vi "Autonomous Independent.vi"   [LabVIEW 2017]
doc: "This VI is called when autonomous begins, and will automatically be terminated when autonomous ends. You can carry out timed or sensor driven robot movement independently without needing to return to the caller."
uses:
  <vilib>/Rock Robotics/WPI/Utilities/WPI_GetSetVariantRefNum.vi
  <vilib>/Rock Robotics/Network Tables/NT Read String.vi
  <vilib>/Rock Robotics/Network Tables/NT Write Numeric Array.vi
  <vilib>/Rock Robotics/WPI/RobotDrive/WPI_RobotDriveArcadeDrive_Standard(NoSaturation).vi
panel:
  # "Be sure to right-click and choose Data Operations>>Make Current Value default if you want to save the array values with the VI"
types:
  T1 = typedef "WPI_JoystickDevRef.ctl" = cluster{"Device":T2}
  T2 = typedef "WPI_JoystickDeviceEnum.ctl" = enum16{"USB 0", "USB 1", "USB 2", "USB 3", "USB 4", "USB 5"}
  T3 = typedef "WPI_MotorControlDeviceRef.ctl" = cluster{"DeviceStatus":errorcluster, "Type":T4, "PWM":cluster{"PWM Channel":T5, "DeadBand":T6}, "CAN":cluster{"Device Number":u8, "SetOutput VI Ref":variant, "GetOutput VI Ref":variant, "Enable VI Ref":variant, "Disable VI Ref":variant, "Data":variant}, "Invert":bool, "DIO PWM":cluster{"PWM \"Enable\" Channel":T5, "DIOChannel":T7, "PWM Rate":dbl}}
  T4 = typedef "WPI_MotorControlType.ctl" = enum16{"PWM", "CAN", "DIO PWM"}
  T5 = typedef "FPGA_DIOPWMChannel.ctl" = enum8{"PWM 0", "PWM 1", "PWM 2", "PWM 3", "PWM 4", "PWM 5", "PWM 6", "PWM 7", "PWM 8", "PWM 9", "PWM MXP 0", "PWM MXP 1", "PWM MXP 2", "PWM MXP 3", "PWM MXP 4", "PWM MXP 5", "PWM MXP 6", "PWM MXP 7", "PWM MXP 8", "PWM MXP 9", "Invalid"}
  T6 = typedef "WPI_PWMDeadband.ctl" = cluster{"Name":string, "maxPositivePwm":i32, "minPositivePwm":i32, "centerPwm":i32, "maxNegativePwm":i32, "minNegativePwm":i32, "angularRange":u16}
  T7 = typedef "FPGA_DIOChannel.ctl" = enum8{"DIO 0", "DIO 1", "DIO 2", "DIO 3", "DIO 4", "DIO 5", "DIO 6", "DIO 7", "DIO 8", "DIO 9", "DIO MXP 0", "DIO MXP 1", "DIO MXP 2", "DIO MXP 3", "DIO MXP 4", "DIO MXP 5", "DIO MXP 6", "DIO MXP 7", "DIO MXP 8", "DIO MXP 9", "DIO MXP 10", "DIO MXP 11", "DIO MXP 12", "DIO MXP 13", "DIO MXP 14", "DIO MXP 15", "SPI Port CS1", "SPI Port CS2", "SPI Port CS3", "SPI Port MISO", "SPI Port MOSI", "Invalid"}
  T8 = typedef "WPI_RobotDriveDevRef.ctl" = cluster{"DevStatus":errorcluster, "Motors[]":T3[], "Square Inputs":bool, "Max Output":dbl}
  T9 = typedef "WPI_SwitchDevRef.ctl" = cluster{"DevStatus":errorcluster, "DIO Channel":T7, "CntIndex":T10, "Normally Closed":bool}
  T10 = typedef "FPGA_CounterCtrSystemIndex.ctl" = enum8{"Ctr 0", "Ctr 1", "Ctr 2", "Ctr 3", "Ctr 4", "Ctr 5", "Ctr 6", "Ctr 7", "Invalid"}
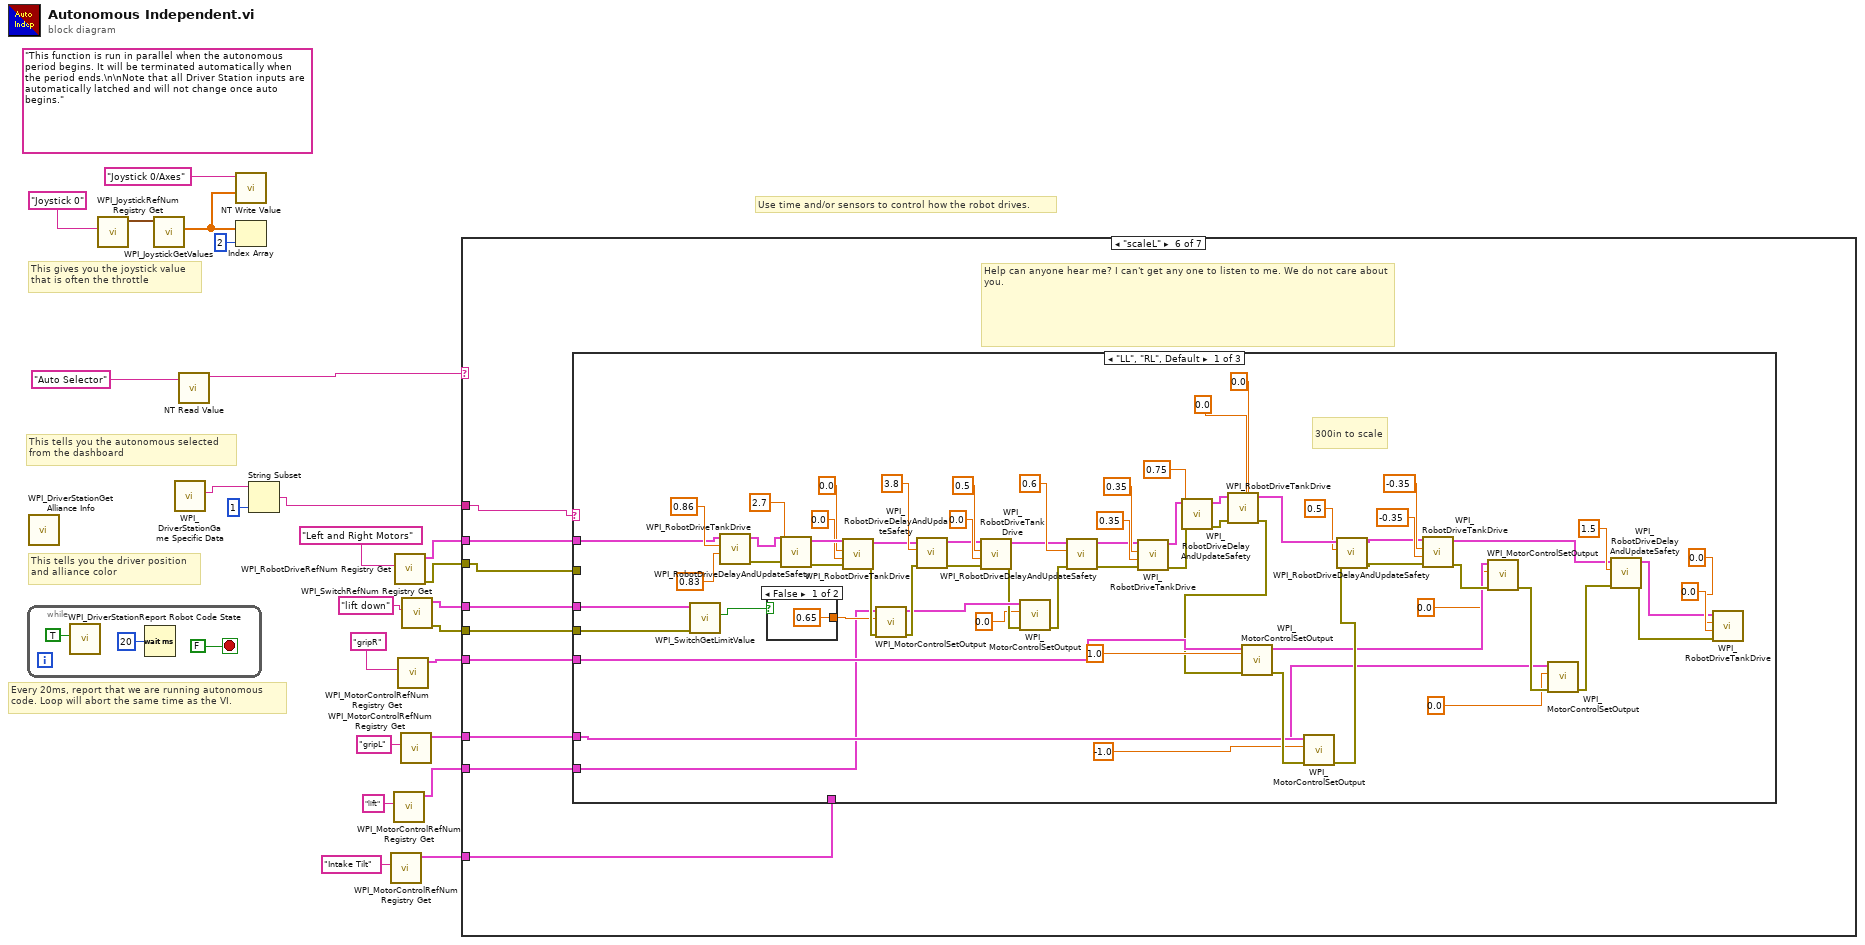
[diagram p0: block diagram]
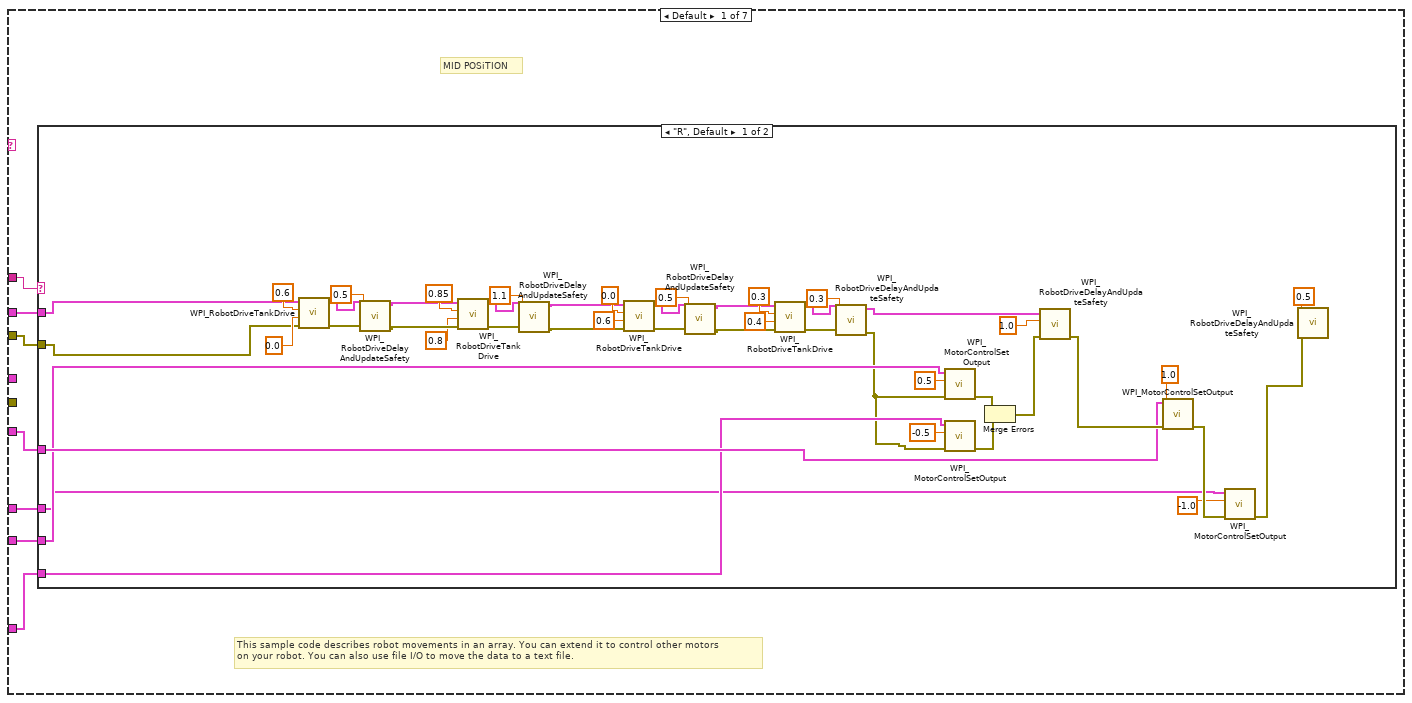
[diagram p2: hidden frame]
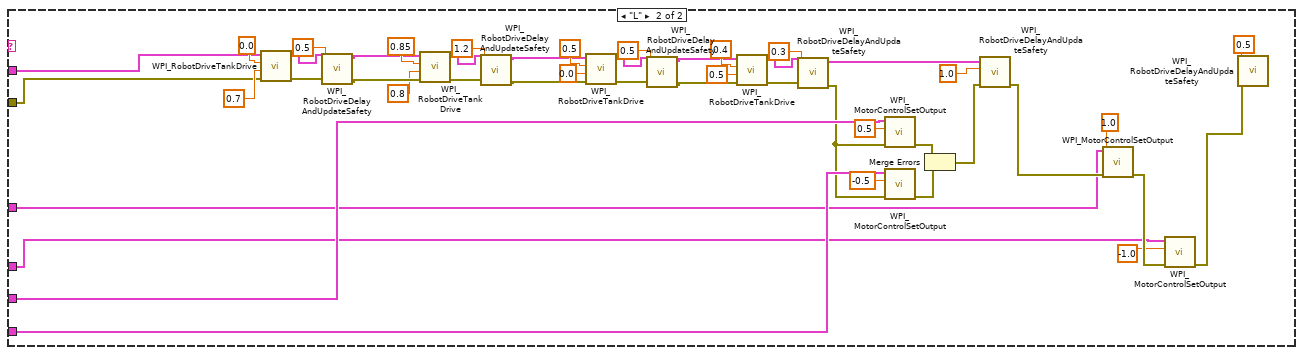
[diagram p3: hidden frame]
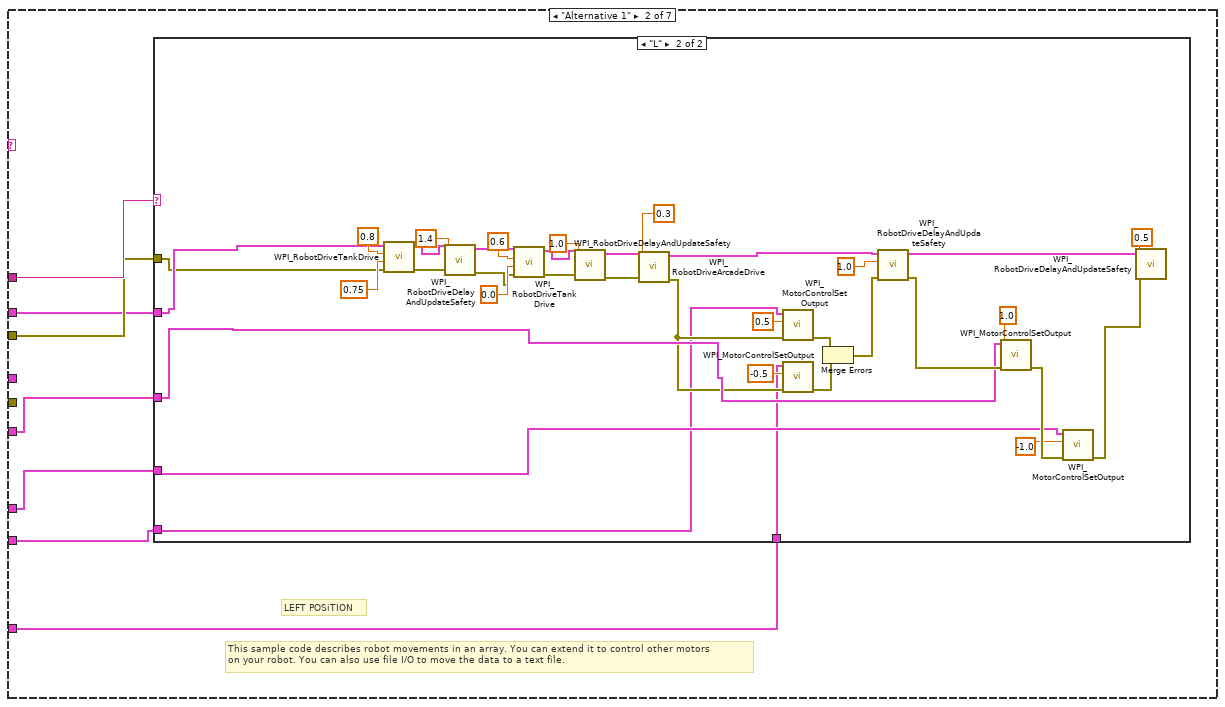
[diagram p4: hidden frame]
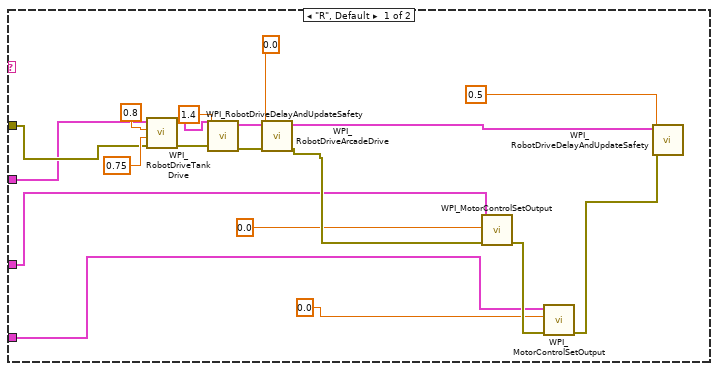
[diagram p5: hidden frame]
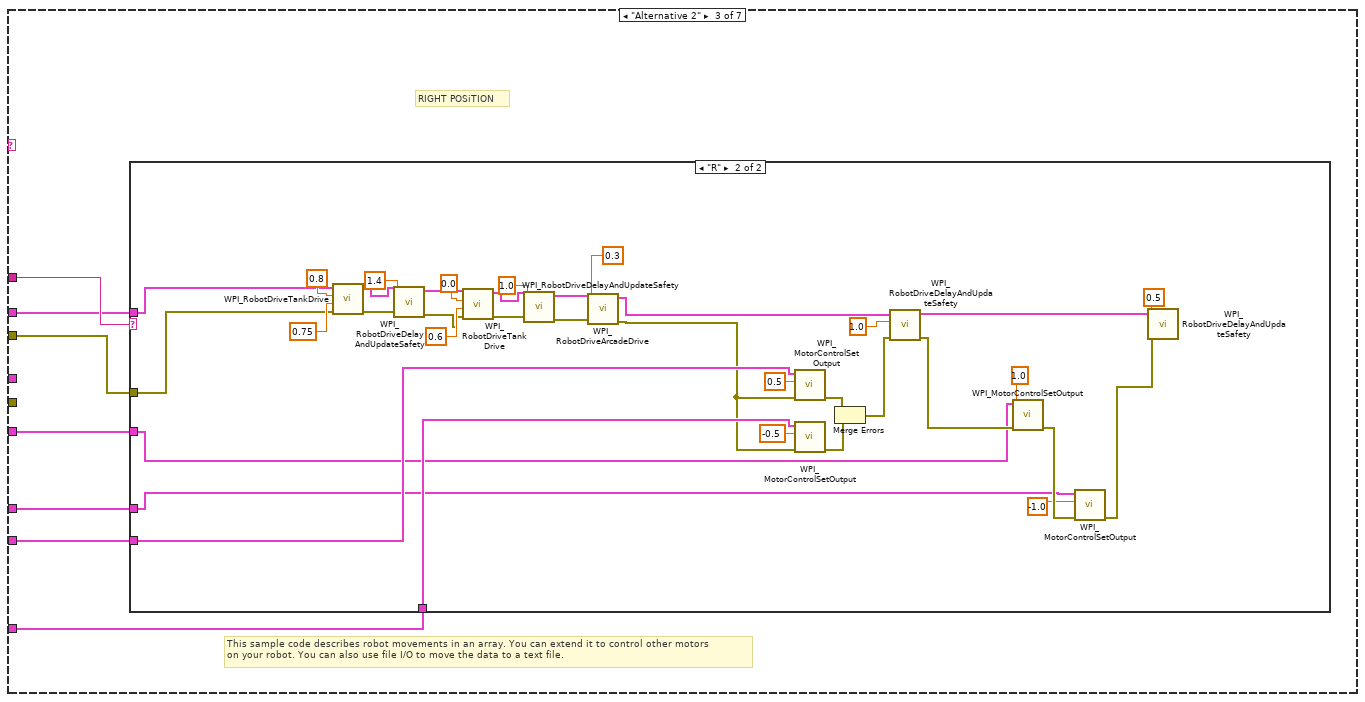
[diagram p6: hidden frame]
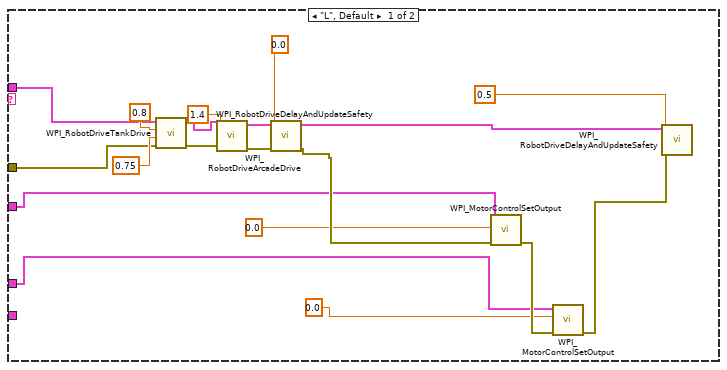
[diagram p7: hidden frame]
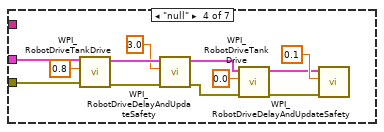
[diagram p8: hidden frame]
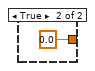
[diagram p10: hidden frame]
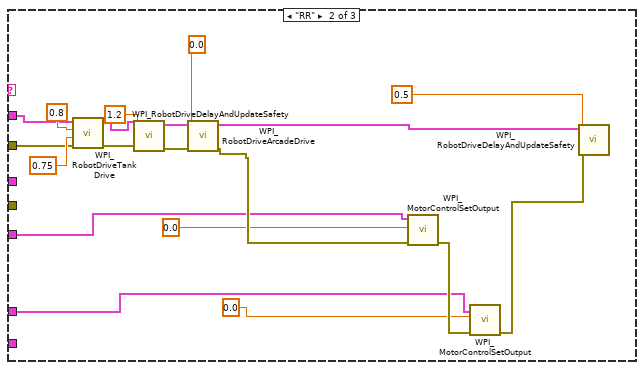
[diagram p11: hidden frame]
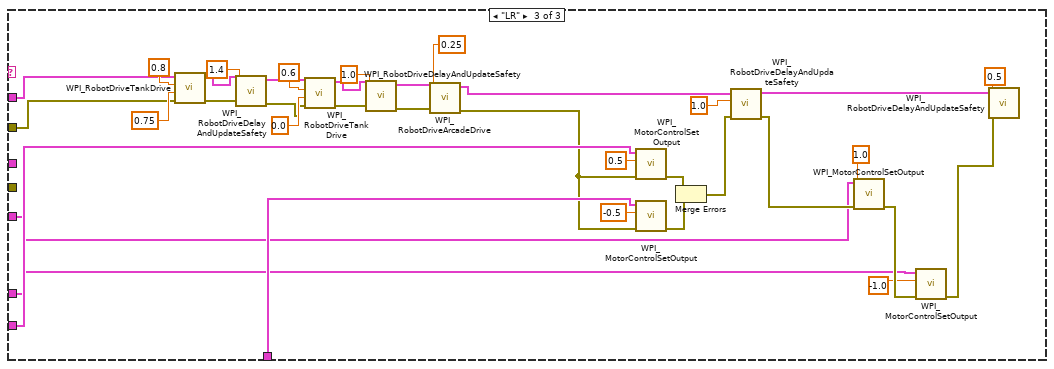
[diagram p12: hidden frame]
diagram:
  (unwired) "This function is run in parallel when the autonomous period begins. It will be terminated automatically when the period ends.\n\nNote that all Driver Station inputs are automatically latched and will not change once auto begins."
  # "This tells you the autonomous selected\nfrom the dashboard"
  # "Every 20ms, report that we are running autonomous\ncode. Loop will abort the same time as the VI."
  # "This gives you the joystick value\nthat is often the throttle"
  # "Use time and/or sensors to control how the robot drives."
  # "This tells you the driver position\nand alliance color"
  n1 = while {
    stop <- FALSE stop-if-true
    n2 = call <vilib>:"WPI_DriverStationReport Robot Code State.vi"("Autonomous"=TRUE) -> ()  [unwired: 10 in, 1 out]
    n3 = Wait (ms)(milliseconds to wait=u32 20) -> ()  [unwired: 1 out]
  }
  n4 = call <vilib>:"WPI_DriverStationGet Alliance Info.vi"() -> ()  [unwired: 12 out]
  n5 = call <vilib>:"WPI_JoystickRefNum Registry Get.vi"("refnum name"="Joystick 0") -> ("JoystickDevRef"=w23:T1)  [unwired: 1 in, 9 out]
  n6 = call <vilib>:"WPI_JoystickGetValues.vi"("JoystickDevRef"=w23) -> ("Axes"=w19:dbl[])  [unwired: 6 in, 4 out]
  n7 = call <vilib>:"WPI_DriverStationGame Specific Data.vi"() -> ("Game Specific Data"=w17:string)  [unwired: 11 in]
  n8 = call-poly <vilib>:"NT Read Value.vi"("Name"="Auto Selector") -> ("String"=w20:string)  [unwired: 9 in, 1 out]
  n9 = call-poly <vilib>:"NT Write Value.vi"("Numeric Array"=w19, "Name"="Joystick 0/Axes") -> ()  [unwired: 9 in, 1 out]
  n10 = Index Array(array=w19, index=2) -> ()  [unwired: 1 out]
  n11 = String Subset(string=w17, length (rest)=1 ("length (rest)")) -> (substring=w15:string)  [unwired: 1 in]
  n12 = call <vilib>:"WPI_MotorControlRefNum Registry Get.vi"("refnum name"="Intake Tilt") -> ("MotorControlDevRef"=w1:T3)  [unwired: 9 in, 1 out]
  n13 = call <vilib>:"WPI_MotorControlRefNum Registry Get.vi"("refnum name"="lift") -> ("MotorControlDevRef"=w3:T3)  [unwired: 9 in, 1 out]
  n14 = call <vilib>:"WPI_RobotDriveRefNum Registry Get.vi"("refnum name"="Left and Right Motors") -> ("error out"=w13:errorcluster, "RobotDriveDevRef"=w8:T8)  [unwired: 1 in, 8 out]
  n15 = call <vilib>:"WPI_MotorControlRefNum Registry Get.vi"("refnum name"="gripR") -> ("MotorControlDevRef"=w11:T3)  [unwired: 9 in, 1 out]
  n16 = call <vilib>:"WPI_MotorControlRefNum Registry Get.vi"("refnum name"="gripL") -> ("MotorControlDevRef"=w9:T3)  [unwired: 9 in, 1 out]
  n17 = call <vilib>:"WPI_SwitchRefNum Registry Get.vi"("refnum name"="lift down") -> ("error out"=w5:errorcluster, "SwitchDevRef"=w4:T9)  [unwired: 9 in]
  n18 = case shown="\"scaleL\"" w20 {
    tunnel: w15 -> [w34 w133 w195 _ _ w271 _]
    tunnel: w13 -> [w33 w132 w194 w261 _ w264 _]
    tunnel: w11 -> [w32 w131 w193 _ _ w268 _]
    tunnel: w9 -> [w31 w130 w192 _ _ w269 _]
    tunnel: w8 -> [w30 w129 w191 w262 _ w270 _]
    tunnel: w5 -> [_ _ _ _ _ w267 _]
    tunnel: w4 -> [_ _ _ _ _ w266 _]
    tunnel: w3 -> [w28 w127 w190 _ _ w265 _]
    tunnel: w1 -> [w29 w128 w189 _ _ w263 _]
    frame Default {
      # "MID POSiTION"
      # "This sample code describes robot movements in an array. You can extend it to control other motors\non your robot. You can also use file I/O to move the data to a text file."
      n19 = case shown="\"R\", Default" w34 {
        tunnel: w33 -> [w75 w95]
        tunnel: w32 -> [w39 w82]
        tunnel: w31 -> [w36 w81]
        tunnel: w30 -> [w53 w94]
        tunnel: w29 -> [w37 w89]
        tunnel: w28 -> [w38 w93]
        frame "R", Default {
          n20 = call <vilib>:"WPI_RobotDriveTankDrive.vi"("error in (no error)"=w75, "Right axis value"=0.0 ("Y axis value"), "Left axis value"=0.6 ("X axis value"), "RobotDriveDevRef"=w53) -> ("error out"=w79:errorcluster, "RobotDriveDevRef"=w78:T8)  [unwired: 5 in, 1 out]
          n21 = call <vilib>:"WPI_RobotDriveDelayAndUpdateSafety.vi"("error in (no error)"=w79, "Delay (s)"=0.5, "RobotDriveDevRef"=w78) -> ("error out"=w69:errorcluster, "RobotDriveDevRef 2"=w70:T8)  [unwired: 7 in]
          n22 = call <vilib>:"WPI_RobotDriveTankDrive.vi"("error in (no error)"=w69, "Right axis value"=0.8, "Left axis value"=0.85 ("X axis value"), "RobotDriveDevRef"=w70) -> ("error out"=w73:errorcluster, "RobotDriveDevRef"=w72:T8)  [unwired: 5 in, 1 out]
          n23 = call <vilib>:"WPI_RobotDriveDelayAndUpdateSafety.vi"("error in (no error)"=w73, "Delay (s)"=1.1, "RobotDriveDevRef"=w72) -> ("error out"=w62:errorcluster, "RobotDriveDevRef 2"=w63:T8)  [unwired: 7 in]
          n24 = call <vilib>:"WPI_RobotDriveTankDrive.vi"("error in (no error)"=w62, "Right axis value"=0.6, "Left axis value"=0.0 ("X axis value"), "RobotDriveDevRef"=w63) -> ("error out"=w66:errorcluster, "RobotDriveDevRef"=w65:T8)  [unwired: 5 in, 1 out]
          n25 = call <vilib>:"WPI_RobotDriveDelayAndUpdateSafety.vi"("error in (no error)"=w66, "Delay (s)"=0.5, "RobotDriveDevRef"=w65) -> ("error out"=w55:errorcluster, "RobotDriveDevRef 2"=w56:T8)  [unwired: 7 in]
          n26 = call <vilib>:"WPI_RobotDriveTankDrive.vi"("error in (no error)"=w55, "Right axis value"=0.4, "Left axis value"=0.3 ("X axis value"), "RobotDriveDevRef"=w56) -> ("error out"=w59:errorcluster, "RobotDriveDevRef"=w58:T8)  [unwired: 5 in, 1 out]
          n27 = call <vilib>:"WPI_RobotDriveDelayAndUpdateSafety.vi"("error in (no error)"=w59, "Delay (s)"=0.3, "RobotDriveDevRef"=w58) -> ("error out"=w35:errorcluster, "RobotDriveDevRef 2"=w40:T8)  [unwired: 7 in]
          n28 = call <vilib>:"WPI_MotorControlSetOutput.vi"("error in (no error)"=w35, "Output"=0.5, "MotorControlDevRef"=w38) -> ("error out"=w43:errorcluster)  [unwired: 6 in, 2 out]
          n29 = call <vilib>:"WPI_MotorControlSetOutput.vi"("error in (no error)"=w35, "Output"=-0.5, "MotorControlDevRef"=w37) -> ("error out"=w44:errorcluster)  [unwired: 6 in, 2 out]
          n30 = Merge Errors(w43, w44) -> (w42:errorcluster)
          n31 = call <vilib>:"WPI_RobotDriveDelayAndUpdateSafety.vi"("error in (no error)"=w42, "Delay (s)"=1.0, "RobotDriveDevRef"=w40) -> ("error out"=w41:errorcluster)  [unwired: 7 in, 1 out]
          n32 = call <vilib>:"WPI_MotorControlSetOutput.vi"("error in (no error)"=w41, "Output"=1.0, "MotorControlDevRef"=w39) -> ("error out"=w51:errorcluster)  [unwired: 6 in, 2 out]
          n33 = call <vilib>:"WPI_MotorControlSetOutput.vi"("error in (no error)"=w51, "Output"=-1.0, "MotorControlDevRef"=w36) -> ("error out"=w50:errorcluster)  [unwired: 6 in, 2 out]
          n34 = call <vilib>:"WPI_RobotDriveDelayAndUpdateSafety.vi"("error in (no error)"=w50, "Delay (s)"=0.5) -> ()  [unwired: 8 in, 2 out]
        }
        frame "L" {
          n35 = call <vilib>:"WPI_RobotDriveTankDrive.vi"("error in (no error)"=w95, "Right axis value"=0.7 ("Y axis value"), "Left axis value"=0.0 ("X axis value"), "RobotDriveDevRef"=w94) -> ("error out"=w122:errorcluster, "RobotDriveDevRef"=w121:T8)  [unwired: 5 in, 1 out]
          n36 = call <vilib>:"WPI_RobotDriveDelayAndUpdateSafety.vi"("error in (no error)"=w122, "Delay (s)"=0.5, "RobotDriveDevRef"=w121) -> ("error out"=w111:errorcluster, "RobotDriveDevRef 2"=w112:T8)  [unwired: 7 in]
          n37 = call <vilib>:"WPI_RobotDriveTankDrive.vi"("error in (no error)"=w111, "Right axis value"=0.8, "Left axis value"=0.85 ("X axis value"), "RobotDriveDevRef"=w112) -> ("error out"=w115:errorcluster, "RobotDriveDevRef"=w114:T8)  [unwired: 5 in, 1 out]
          n38 = call <vilib>:"WPI_RobotDriveDelayAndUpdateSafety.vi"("error in (no error)"=w115, "Delay (s)"=1.2, "RobotDriveDevRef"=w114) -> ("error out"=w104:errorcluster, "RobotDriveDevRef 2"=w105:T8)  [unwired: 7 in]
          n39 = call <vilib>:"WPI_RobotDriveTankDrive.vi"("error in (no error)"=w104, "Right axis value"=0.0, "Left axis value"=0.5 ("X axis value"), "RobotDriveDevRef"=w105) -> ("error out"=w108:errorcluster, "RobotDriveDevRef"=w107:T8)  [unwired: 5 in, 1 out]
          n40 = call <vilib>:"WPI_RobotDriveDelayAndUpdateSafety.vi"("error in (no error)"=w108, "Delay (s)"=0.5, "RobotDriveDevRef"=w107) -> ("error out"=w97:errorcluster, "RobotDriveDevRef 2"=w98:T8)  [unwired: 7 in]
          n41 = call <vilib>:"WPI_RobotDriveTankDrive.vi"("error in (no error)"=w97, "Right axis value"=0.5, "Left axis value"=0.4 ("X axis value"), "RobotDriveDevRef"=w98) -> ("error out"=w101:errorcluster, "RobotDriveDevRef"=w100:T8)  [unwired: 5 in, 1 out]
          n42 = call <vilib>:"WPI_RobotDriveDelayAndUpdateSafety.vi"("error in (no error)"=w101, "Delay (s)"=0.3, "RobotDriveDevRef"=w100) -> ("error out"=w87:errorcluster, "RobotDriveDevRef 2"=w91:T8)  [unwired: 7 in]
          n43 = call <vilib>:"WPI_MotorControlSetOutput.vi"("error in (no error)"=w87, "Output"=0.5, "MotorControlDevRef"=w93) -> ("error out"=w85:errorcluster)  [unwired: 6 in, 2 out]
          n44 = call <vilib>:"WPI_MotorControlSetOutput.vi"("error in (no error)"=w87, "Output"=-0.5, "MotorControlDevRef"=w89) -> ("error out"=w86:errorcluster)  [unwired: 6 in, 2 out]
          n45 = Merge Errors(w85, w86) -> (w84:errorcluster)
          n46 = call <vilib>:"WPI_RobotDriveDelayAndUpdateSafety.vi"("error in (no error)"=w84, "Delay (s)"=1.0, "RobotDriveDevRef"=w91) -> ("error out"=w83:errorcluster)  [unwired: 7 in, 1 out]
          n47 = call <vilib>:"WPI_MotorControlSetOutput.vi"("error in (no error)"=w83, "Output"=1.0, "MotorControlDevRef"=w82) -> ("error out"=w124:errorcluster)  [unwired: 6 in, 2 out]
          n48 = call <vilib>:"WPI_MotorControlSetOutput.vi"("error in (no error)"=w124, "Output"=-1.0, "MotorControlDevRef"=w81) -> ("error out"=w123:errorcluster)  [unwired: 6 in, 2 out]
          n49 = call <vilib>:"WPI_RobotDriveDelayAndUpdateSafety.vi"("error in (no error)"=w123, "Delay (s)"=0.5) -> ()  [unwired: 8 in, 2 out]
        }
      }
    }
    frame "Alternative 1" {
      # "LEFT POSiTION"
      # "This sample code describes robot movements in an array. You can extend it to control other motors\non your robot. You can also use file I/O to move the data to a text file."
      n50 = case shown="\"L\"" w133 {
        tunnel: w132 -> [w137 w172]
        tunnel: w131 -> [w136 w158]
        tunnel: w130 -> [w135 w156]
        tunnel: w129 -> [w134 w173]
        tunnel: w128 -> [_ w155]
        tunnel: w127 -> [_ w154]
        frame "R", Default {
          n51 = call <vilib>:"WPI_RobotDriveTankDrive.vi"("error in (no error)"=w137, "Right axis value"=0.75 ("Y axis value"), "Left axis value"=0.8 ("X axis value"), "RobotDriveDevRef"=w134) -> ("error out"=w143:errorcluster, "RobotDriveDevRef"=w142:T8)  [unwired: 5 in, 1 out]
          n52 = call <vilib>:"WPI_RobotDriveDelayAndUpdateSafety.vi"("error in (no error)"=w143, "Delay (s)"=1.4, "RobotDriveDevRef"=w142) -> ("error out"=w151:errorcluster, "RobotDriveDevRef 2"=w150:T8)  [unwired: 7 in]
          n53 = call-poly <vilib>:"WPI_RobotDriveArcadeDrive.vi"("error in (no error)"=w151, "Y axis value"=0.0, "RobotDriveDevRef"=w150) -> ("error out"=w145:errorcluster, "RobotDriveDevRef"=w148:T8)  [unwired: 6 in, 1 out]
          n54 = call <vilib>:"WPI_MotorControlSetOutput.vi"("error in (no error)"=w145, "Output"=0.0, "MotorControlDevRef"=w136) -> ("error out"=w146:errorcluster)  [unwired: 6 in, 2 out]
          n55 = call <vilib>:"WPI_MotorControlSetOutput.vi"("error in (no error)"=w146, "Output"=0.0, "MotorControlDevRef"=w135) -> ("error out"=w144:errorcluster)  [unwired: 6 in, 2 out]
          n56 = call <vilib>:"WPI_RobotDriveDelayAndUpdateSafety.vi"("error in (no error)"=w144, "Delay (s)"=0.5, "RobotDriveDevRef"=w148) -> ()  [unwired: 7 in, 2 out]
        }
        frame "L" {
          n57 = call <vilib>:"WPI_RobotDriveTankDrive.vi"("error in (no error)"=w172, "Right axis value"=0.75 ("Y axis value"), "Left axis value"=0.8 ("X axis value"), "RobotDriveDevRef"=w173) -> ("error out"=w186:errorcluster, "RobotDriveDevRef"=w185:T8)  [unwired: 5 in, 1 out]
          n58 = call <vilib>:"WPI_RobotDriveDelayAndUpdateSafety.vi"("error in (no error)"=w186, "Delay (s)"=1.4, "RobotDriveDevRef"=w185) -> ("error out"=w176:errorcluster, "RobotDriveDevRef 2"=w177:T8)  [unwired: 7 in]
          n59 = call <vilib>:"WPI_RobotDriveTankDrive.vi"("error in (no error)"=w176, "Right axis value"=0.0 ("Y axis value"), "Left axis value"=0.6 ("X axis value"), "RobotDriveDevRef"=w177) -> ("error out"=w181:errorcluster, "RobotDriveDevRef"=w180:T8)  [unwired: 5 in, 1 out]
          n60 = call <vilib>:"WPI_RobotDriveDelayAndUpdateSafety.vi"("error in (no error)"=w181, "Delay (s)"=1.0, "RobotDriveDevRef"=w180) -> ("error out"=w174:errorcluster, "RobotDriveDevRef 2"=w175:T8)  [unwired: 7 in]
          n61 = call-poly <vilib>:"WPI_RobotDriveArcadeDrive.vi"("error in (no error)"=w174, "Y axis value"=0.3, "RobotDriveDevRef"=w175) -> ("error out"=w157:errorcluster, "RobotDriveDevRef"=w159:T8)  [unwired: 6 in, 1 out]
          n62 = call <vilib>:"WPI_MotorControlSetOutput.vi"("error in (no error)"=w157, "Output"=0.5, "MotorControlDevRef"=w154) -> ("error out"=w162:errorcluster)  [unwired: 6 in, 2 out]
          n63 = call <vilib>:"WPI_MotorControlSetOutput.vi"("error in (no error)"=w157, "Output"=-0.5, "MotorControlDevRef"=w155) -> ("error out"=w163:errorcluster)  [unwired: 6 in, 2 out]
          n64 = Merge Errors(w162, w163) -> (w161:errorcluster)
          n65 = call <vilib>:"WPI_RobotDriveDelayAndUpdateSafety.vi"("error in (no error)"=w161, "Delay (s)"=1.0, "RobotDriveDevRef"=w159) -> ("error out"=w160:errorcluster, "RobotDriveDevRef 2"=w153:T8)  [unwired: 7 in]
          n66 = call <vilib>:"WPI_MotorControlSetOutput.vi"("error in (no error)"=w160, "Output"=1.0, "MotorControlDevRef"=w158) -> ("error out"=w170:errorcluster)  [unwired: 6 in, 2 out]
          n67 = call <vilib>:"WPI_MotorControlSetOutput.vi"("error in (no error)"=w170, "Output"=-1.0, "MotorControlDevRef"=w156) -> ("error out"=w169:errorcluster)  [unwired: 6 in, 2 out]
          n68 = call <vilib>:"WPI_RobotDriveDelayAndUpdateSafety.vi"("error in (no error)"=w169, "Delay (s)"=0.5, "RobotDriveDevRef"=w153) -> ()  [unwired: 7 in, 2 out]
        }
      }
    }
    frame "Alternative 2" {
      # "RIGHT POSiTION"
      # "This sample code describes robot movements in an array. You can extend it to control other motors\non your robot. You can also use file I/O to move the data to a text file."
      n69 = case shown="\"R\"" w195 {
        tunnel: w194 -> [w197 w234]
        tunnel: w193 -> [w198 w217]
        tunnel: w192 -> [w199 w216]
        tunnel: w191 -> [w196 w235]
        tunnel: w190 -> [_ w219]
        tunnel: w189 -> [_ w218]
        frame "L", Default {
          n70 = call <vilib>:"WPI_RobotDriveTankDrive.vi"("error in (no error)"=w197, "Right axis value"=0.75 ("Y axis value"), "Left axis value"=0.8 ("X axis value"), "RobotDriveDevRef"=w196) -> ("error out"=w205:errorcluster, "RobotDriveDevRef"=w204:T8)  [unwired: 5 in, 1 out]
          n71 = call <vilib>:"WPI_RobotDriveDelayAndUpdateSafety.vi"("error in (no error)"=w205, "Delay (s)"=1.4, "RobotDriveDevRef"=w204) -> ("error out"=w213:errorcluster, "RobotDriveDevRef 2"=w212:T8)  [unwired: 7 in]
          n72 = call-poly <vilib>:"WPI_RobotDriveArcadeDrive.vi"("error in (no error)"=w213, "Y axis value"=0.0, "RobotDriveDevRef"=w212) -> ("error out"=w207:errorcluster, "RobotDriveDevRef"=w210:T8)  [unwired: 6 in, 1 out]
          n73 = call <vilib>:"WPI_MotorControlSetOutput.vi"("error in (no error)"=w207, "Output"=0.0, "MotorControlDevRef"=w198) -> ("error out"=w208:errorcluster)  [unwired: 6 in, 2 out]
          n74 = call <vilib>:"WPI_MotorControlSetOutput.vi"("error in (no error)"=w208, "Output"=0.0, "MotorControlDevRef"=w199) -> ("error out"=w206:errorcluster)  [unwired: 6 in, 2 out]
          n75 = call <vilib>:"WPI_RobotDriveDelayAndUpdateSafety.vi"("error in (no error)"=w206, "Delay (s)"=0.5, "RobotDriveDevRef"=w210) -> ()  [unwired: 7 in, 2 out]
        }
        frame "R" {
          n76 = call <vilib>:"WPI_RobotDriveTankDrive.vi"("error in (no error)"=w234, "Right axis value"=0.75 ("Y axis value"), "Left axis value"=0.8 ("X axis value"), "RobotDriveDevRef"=w235) -> ("error out"=w248:errorcluster, "RobotDriveDevRef"=w247:T8)  [unwired: 5 in, 1 out]
          n77 = call <vilib>:"WPI_RobotDriveDelayAndUpdateSafety.vi"("error in (no error)"=w248, "Delay (s)"=1.4, "RobotDriveDevRef"=w247) -> ("error out"=w238:errorcluster, "RobotDriveDevRef 2"=w239:T8)  [unwired: 7 in]
          n78 = call <vilib>:"WPI_RobotDriveTankDrive.vi"("error in (no error)"=w238, "Right axis value"=0.6 ("Y axis value"), "Left axis value"=0.0 ("X axis value"), "RobotDriveDevRef"=w239) -> ("error out"=w243:errorcluster, "RobotDriveDevRef"=w242:T8)  [unwired: 5 in, 1 out]
          n79 = call <vilib>:"WPI_RobotDriveDelayAndUpdateSafety.vi"("error in (no error)"=w243, "Delay (s)"=1.0, "RobotDriveDevRef"=w242) -> ("error out"=w236:errorcluster, "RobotDriveDevRef 2"=w237:T8)  [unwired: 7 in]
          n80 = call-poly <vilib>:"WPI_RobotDriveArcadeDrive.vi"("error in (no error)"=w236, "Y axis value"=0.3, "RobotDriveDevRef"=w237) -> ("error out"=w215:errorcluster, "RobotDriveDevRef"=w221:T8)  [unwired: 6 in, 1 out]
          n81 = call <vilib>:"WPI_MotorControlSetOutput.vi"("error in (no error)"=w215, "Output"=0.5, "MotorControlDevRef"=w219) -> ("error out"=w224:errorcluster)  [unwired: 6 in, 2 out]
          n82 = call <vilib>:"WPI_MotorControlSetOutput.vi"("error in (no error)"=w215, "Output"=-0.5, "MotorControlDevRef"=w218) -> ("error out"=w225:errorcluster)  [unwired: 6 in, 2 out]
          n83 = Merge Errors(w224, w225) -> (w223:errorcluster)
          n84 = call <vilib>:"WPI_RobotDriveDelayAndUpdateSafety.vi"("error in (no error)"=w223, "Delay (s)"=1.0, "RobotDriveDevRef"=w221) -> ("error out"=w222:errorcluster, "RobotDriveDevRef 2"=w220:T8)  [unwired: 7 in]
          n85 = call <vilib>:"WPI_MotorControlSetOutput.vi"("error in (no error)"=w222, "Output"=1.0, "MotorControlDevRef"=w217) -> ("error out"=w232:errorcluster)  [unwired: 6 in, 2 out]
          n86 = call <vilib>:"WPI_MotorControlSetOutput.vi"("error in (no error)"=w232, "Output"=-1.0, "MotorControlDevRef"=w216) -> ("error out"=w231:errorcluster)  [unwired: 6 in, 2 out]
          n87 = call <vilib>:"WPI_RobotDriveDelayAndUpdateSafety.vi"("error in (no error)"=w231, "Delay (s)"=0.5, "RobotDriveDevRef"=w220) -> ()  [unwired: 7 in, 2 out]
        }
      }
    }
    frame "null" {
      n88 = call <vilib>:"WPI_RobotDriveTankDrive.vi"("error in (no error)"=w261, "Left axis value"=0.8, "RobotDriveDevRef"=w262) -> ("error out"=w258:errorcluster, "RobotDriveDevRef"=w259:T8)  [unwired: 6 in, 1 out]
      n89 = call <vilib>:"WPI_RobotDriveDelayAndUpdateSafety.vi"("error in (no error)"=w258, "Delay (s)"=3.0, "RobotDriveDevRef"=w259) -> ("error out"=w251:errorcluster, "RobotDriveDevRef 2"=w252:T8)  [unwired: 7 in]
      n90 = call <vilib>:"WPI_RobotDriveTankDrive.vi"("error in (no error)"=w251, "Left axis value"=0.0, "RobotDriveDevRef"=w252) -> ("error out"=w255:errorcluster, "RobotDriveDevRef"=w254:T8)  [unwired: 6 in, 1 out]
      n91 = call <vilib>:"WPI_RobotDriveDelayAndUpdateSafety.vi"("error in (no error)"=w255, "Delay (s)"=0.1, "RobotDriveDevRef"=w254) -> ()  [unwired: 7 in, 2 out]
    }
    frame "drive" {
    }
    frame "scaleL" {
      # "Help can anyone hear me? I can't get any one to listen to me. We do not care about you."
      n92 = case shown="\"LL\", \"RL\", Default" w271 {
        tunnel: w270 -> [w328 w342 w388]
        tunnel: w269 -> [w308 w340 w359]
        tunnel: w268 -> [w309 w341 w360]
        tunnel: w267 -> [w305 _ _]
        tunnel: w266 -> [w304 _ _]
        tunnel: w265 -> [w303 _ w363]
        tunnel: w264 -> [_ w343 w387]
        tunnel: w263 -> [_ _ w362]
        frame "LL", "RL", Default {
          # "300in to scale"
          n93 = call <vilib>:"WPI_SwitchGetLimitValue.vi"("error in (no error)"=w305, "SwitchDevRef"=w304) -> ("Switch Pressed"=w306:bool)  [unwired: 7 in, 2 out]
          n94 = call <vilib>:"WPI_RobotDriveTankDrive.vi"("Right axis value"=0.83 ("Y axis value"), "Left axis value"=0.86 ("X axis value"), "RobotDriveDevRef"=w328) -> ("error out"=w334:errorcluster, "RobotDriveDevRef"=w333:T8)  [unwired: 6 in, 1 out]
          n95 = case shown="False" w306 {
            tunnel: [0.65 ("Output") 0.0 ("Output")] -> w307
            frame False {
            }
            frame True {
            }
          }
          n96 = call <vilib>:"WPI_RobotDriveDelayAndUpdateSafety.vi"("error in (no error)"=w334, "Delay (s)"=2.7, "RobotDriveDevRef"=w333) -> ("error out"=w326:errorcluster, "RobotDriveDevRef 2"=w327:T8)  [unwired: 7 in]
          n97 = call <vilib>:"WPI_RobotDriveTankDrive.vi"("error in (no error)"=w326, "Right axis value"=0.0, "Left axis value"=0.0, "RobotDriveDevRef"=w327) -> ("error out"=w323:errorcluster, "RobotDriveDevRef"=w321:T8)  [unwired: 5 in, 1 out]
          n98 = call <vilib>:"WPI_MotorControlSetOutput.vi"("error in (no error)"=w323, "Output"=w307, "MotorControlDevRef"=w303) -> ("error out"=w320:errorcluster, "MotorControlDevRef"=w302:T3)  [unwired: 6 in, 1 out]
          n99 = call <vilib>:"WPI_RobotDriveDelayAndUpdateSafety.vi"("error in (no error)"=w320, "Delay (s)"=3.8, "RobotDriveDevRef"=w321) -> ("error out"=w314:errorcluster, "RobotDriveDevRef 2"=w315:T8)  [unwired: 7 in]
          n100 = call <vilib>:"WPI_RobotDriveTankDrive.vi"("error in (no error)"=w314, "Right axis value"=0.0, "Left axis value"=0.5, "RobotDriveDevRef"=w315) -> ("error out"=w301:errorcluster, "RobotDriveDevRef"=w316:T8)  [unwired: 5 in, 1 out]
          n101 = call <vilib>:"WPI_MotorControlSetOutput.vi"("error in (no error)"=w301, "Output"=0.0, "MotorControlDevRef"=w302) -> ("error out"=w300:errorcluster)  [unwired: 6 in, 2 out]
          n102 = call <vilib>:"WPI_RobotDriveDelayAndUpdateSafety.vi"("error in (no error)"=w300, "Delay (s)"=0.6, "RobotDriveDevRef"=w316) -> ("error out"=w310:errorcluster, "RobotDriveDevRef 2"=w311:T8)  [unwired: 7 in]
          n103 = call <vilib>:"WPI_RobotDriveTankDrive.vi"("error in (no error)"=w310, "Right axis value"=0.35, "Left axis value"=0.35, "RobotDriveDevRef"=w311) -> ("error out"=w284:errorcluster, "RobotDriveDevRef"=w285:T8)  [unwired: 5 in, 1 out]
          n104 = call <vilib>:"WPI_RobotDriveDelayAndUpdateSafety.vi"("error in (no error)"=w284, "Delay (s)"=0.75, "RobotDriveDevRef"=w285) -> ("error out"=w282:errorcluster, "RobotDriveDevRef 2"=w283:T8)  [unwired: 7 in]
          n105 = call <vilib>:"WPI_RobotDriveTankDrive.vi"("error in (no error)"=w282, "Right axis value"=0.0, "Left axis value"=0.0, "RobotDriveDevRef"=w283) -> ("error out"=w281:errorcluster, "RobotDriveDevRef"=w280:T8)  [unwired: 5 in, 1 out]
          n106 = call <vilib>:"WPI_MotorControlSetOutput.vi"("error in (no error)"=w281, "Output"=1.0, "MotorControlDevRef"=w309) -> ("error out"=w336:errorcluster, "MotorControlDevRef"=w292:T3)  [unwired: 6 in, 1 out]
          n107 = call <vilib>:"WPI_MotorControlSetOutput.vi"("error in (no error)"=w336, "Output"=-1.0, "MotorControlDevRef"=w308) -> ("error out"=w335:errorcluster, "MotorControlDevRef"=w291:T3)  [unwired: 6 in, 1 out]
          n108 = call <vilib>:"WPI_RobotDriveDelayAndUpdateSafety.vi"("error in (no error)"=w335, "Delay (s)"=0.5, "RobotDriveDevRef"=w280) -> ("error out"=w295:errorcluster, "RobotDriveDevRef 2"=w296:T8)  [unwired: 7 in]
          n109 = call <vilib>:"WPI_RobotDriveTankDrive.vi"("error in (no error)"=w295, "Right axis value"=-0.35, "Left axis value"=-0.35, "RobotDriveDevRef"=w296) -> ("error out"=w293:errorcluster, "RobotDriveDevRef"=w277:T8)  [unwired: 5 in, 1 out]
          n110 = call <vilib>:"WPI_MotorControlSetOutput.vi"("error in (no error)"=w293, "Output"=0.0, "MotorControlDevRef"=w292) -> ("error out"=w294:errorcluster)  [unwired: 6 in, 2 out]
          n111 = call <vilib>:"WPI_MotorControlSetOutput.vi"("error in (no error)"=w294, "Output"=0.0, "MotorControlDevRef"=w291) -> ("error out"=w276:errorcluster)  [unwired: 6 in, 2 out]
          n112 = call <vilib>:"WPI_RobotDriveDelayAndUpdateSafety.vi"("error in (no error)"=w276, "Delay (s)"=1.5, "RobotDriveDevRef"=w277) -> ("error out"=w272:errorcluster, "RobotDriveDevRef 2"=w273:T8)  [unwired: 7 in]
          n113 = call <vilib>:"WPI_RobotDriveTankDrive.vi"("error in (no error)"=w272, "Right axis value"=0.0, "Left axis value"=0.0, "RobotDriveDevRef"=w273) -> ()  [unwired: 5 in, 3 out]
        }
        frame "RR" {
          n114 = call <vilib>:"WPI_RobotDriveTankDrive.vi"("error in (no error)"=w343, "Right axis value"=0.75 ("Y axis value"), "Left axis value"=0.8 ("X axis value"), "RobotDriveDevRef"=w342) -> ("error out"=w349:errorcluster, "RobotDriveDevRef"=w348:T8)  [unwired: 5 in, 1 out]
          n115 = call <vilib>:"WPI_RobotDriveDelayAndUpdateSafety.vi"("error in (no error)"=w349, "Delay (s)"=1.2, "RobotDriveDevRef"=w348) -> ("error out"=w357:errorcluster, "RobotDriveDevRef 2"=w356:T8)  [unwired: 7 in]
          n116 = call-poly <vilib>:"WPI_RobotDriveArcadeDrive.vi"("error in (no error)"=w357, "Y axis value"=0.0, "RobotDriveDevRef"=w356) -> ("error out"=w351:errorcluster, "RobotDriveDevRef"=w354:T8)  [unwired: 6 in, 1 out]
          n117 = call <vilib>:"WPI_MotorControlSetOutput.vi"("error in (no error)"=w351, "Output"=0.0, "MotorControlDevRef"=w341) -> ("error out"=w352:errorcluster)  [unwired: 6 in, 2 out]
          n118 = call <vilib>:"WPI_MotorControlSetOutput.vi"("error in (no error)"=w352, "Output"=0.0, "MotorControlDevRef"=w340) -> ("error out"=w350:errorcluster)  [unwired: 6 in, 2 out]
          n119 = call <vilib>:"WPI_RobotDriveDelayAndUpdateSafety.vi"("error in (no error)"=w350, "Delay (s)"=0.5, "RobotDriveDevRef"=w354) -> ()  [unwired: 7 in, 2 out]
        }
        frame "LR" {
          n120 = call <vilib>:"WPI_RobotDriveTankDrive.vi"("error in (no error)"=w387, "Right axis value"=0.75 ("Y axis value"), "Left axis value"=0.8 ("X axis value"), "RobotDriveDevRef"=w388) -> ("error out"=w392:errorcluster, "RobotDriveDevRef"=w391:T8)  [unwired: 5 in, 1 out]
          n121 = call <vilib>:"WPI_RobotDriveDelayAndUpdateSafety.vi"("error in (no error)"=w392, "Delay (s)"=1.4, "RobotDriveDevRef"=w391) -> ("error out"=w380:errorcluster, "RobotDriveDevRef 2"=w381:T8)  [unwired: 7 in]
          n122 = call <vilib>:"WPI_RobotDriveTankDrive.vi"("error in (no error)"=w380, "Right axis value"=0.0 ("Y axis value"), "Left axis value"=0.6 ("X axis value"), "RobotDriveDevRef"=w381) -> ("error out"=w385:errorcluster, "RobotDriveDevRef"=w384:T8)  [unwired: 5 in, 1 out]
          n123 = call <vilib>:"WPI_RobotDriveDelayAndUpdateSafety.vi"("error in (no error)"=w385, "Delay (s)"=1.0, "RobotDriveDevRef"=w384) -> ("error out"=w378:errorcluster, "RobotDriveDevRef 2"=w379:T8)  [unwired: 7 in]
          n124 = call-poly <vilib>:"WPI_RobotDriveArcadeDrive.vi"("error in (no error)"=w378, "Y axis value"=0.25, "RobotDriveDevRef"=w379) -> ("error out"=w361:errorcluster, "RobotDriveDevRef"=w365:T8)  [unwired: 6 in, 1 out]
          n125 = call <vilib>:"WPI_MotorControlSetOutput.vi"("error in (no error)"=w361, "Output"=0.5, "MotorControlDevRef"=w363) -> ("error out"=w368:errorcluster)  [unwired: 6 in, 2 out]
          n126 = call <vilib>:"WPI_MotorControlSetOutput.vi"("error in (no error)"=w361, "Output"=-0.5, "MotorControlDevRef"=w362) -> ("error out"=w369:errorcluster)  [unwired: 6 in, 2 out]
          n127 = Merge Errors(w368, w369) -> (w367:errorcluster)
          n128 = call <vilib>:"WPI_RobotDriveDelayAndUpdateSafety.vi"("error in (no error)"=w367, "Delay (s)"=1.0, "RobotDriveDevRef"=w365) -> ("error out"=w366:errorcluster, "RobotDriveDevRef 2"=w364:T8)  [unwired: 7 in]
          n129 = call <vilib>:"WPI_MotorControlSetOutput.vi"("error in (no error)"=w366, "Output"=1.0, "MotorControlDevRef"=w360) -> ("error out"=w376:errorcluster)  [unwired: 6 in, 2 out]
          n130 = call <vilib>:"WPI_MotorControlSetOutput.vi"("error in (no error)"=w376, "Output"=-1.0, "MotorControlDevRef"=w359) -> ("error out"=w375:errorcluster)  [unwired: 6 in, 2 out]
          n131 = call <vilib>:"WPI_RobotDriveDelayAndUpdateSafety.vi"("error in (no error)"=w375, "Delay (s)"=0.5, "RobotDriveDevRef"=w364) -> ()  [unwired: 7 in, 2 out]
        }
      }
    }
    frame "scaleR" {
    }
  }
